vi "4155C Output-FPP.vi"(0 "VISA resource name in":refnum<visa-resource-name>="GPIB0::14::INSTR", 2 "Gate":T4={"Gate Start"=0.0, "Gate Stop"=2.0, "Gate Step"=1.0, "Gate Compliance"=0.0001, "Gate PComp"=0.0, "Range mode"=0, "Range"=6} {"Range" max=11 scale=0.0..11.0; "Range mode" items=["Auto", "Limited", "Fixed"]; "Gate PComp" format="%^.2e"; "Gate Compliance" format="%^.2e"; "Gate Step" format="%^.4e"; "Gate Stop" format="%^.4e"; "Gate Start" format="%^.4e"}, 3 "Drain":T5={"Drain Start"=0.0, "Drain Stop"=2.0, "Drain Compliance"=0.0001, "Drain Step (linear only)"=1.0, "Drain PComp"=0.0, "Range mode"=0, "Range"=6} {"Range" max=11 scale=0.0..11.0; "Range mode" items=["Auto", "Limited", "Fixed"]; "Drain PComp" format="%^.2e"; "Drain Step (linear only)" format="%^.4e"; "Drain Compliance" format="%^.2e"; "Drain Stop" format="%^.4e"; "Drain Start" format="%^.4e"}, 5 "Timings":T3={"integration time"=0, "Short/Long integration time"=0.00064, "hold time (sec)"=0.0, "delay time (sec)"=0.0, "Step Time (0 disables)"=0.0, "sweep method"=0, "Pulse period"=0.005, "Base voltage"=0.0, "Pulse width"=0.0005} {"Pulse width" min=0.0005 max=0.1 step=0.0001 format="%.4f"; "Base voltage" format="%^.4e"; "Pulse period" min=0.005 max=1.0 step=0.0001 format="%.4f"; "sweep method" items=["Continuous", "Pulsed"]; "Step Time (0 disables)" format="%.2f"; "delay time (sec)" format="%.4f"; "hold time (sec)" format="%.4f"; "Short/Long integration time" format="%^.0e"; "integration time" scale=0.0..2.0}, 6 "error in (no error)":errorcluster, 10 "sweep mode":u16(ring) items=["Single", "Double"], 12 "Panel controls":T2={"Emergency Stop"=refnum, "OutputGraph Max"=1e-05, "Text/Graph (text=false)"=FALSE} {"OutputGraph Max" format="%.2e"}) -> (16 "VD":dbl[](array[numeric]) format="%.2f", 17 "Outparams":T1={"V2 Start"=0.0, "V2 Step"=0.0, "Number of points"=1} {"V2 Step" format="%.2f"; "V2 Start" format="%^.4e"}, 20 "VISA Resource Name out":refnum<visa-resource-name>, 21 "Vprobe2":dbl[](array[numeric]) format="%.2f", 22 "ID":dbl[](array[numeric]) format="%.2f", 23 "IG":dbl[](array[numeric]) format="%.2f", 25 "Vprobe1":dbl[](array[numeric]) format="%.2f", 26 "error out":errorcluster)   [LabVIEW 2016]
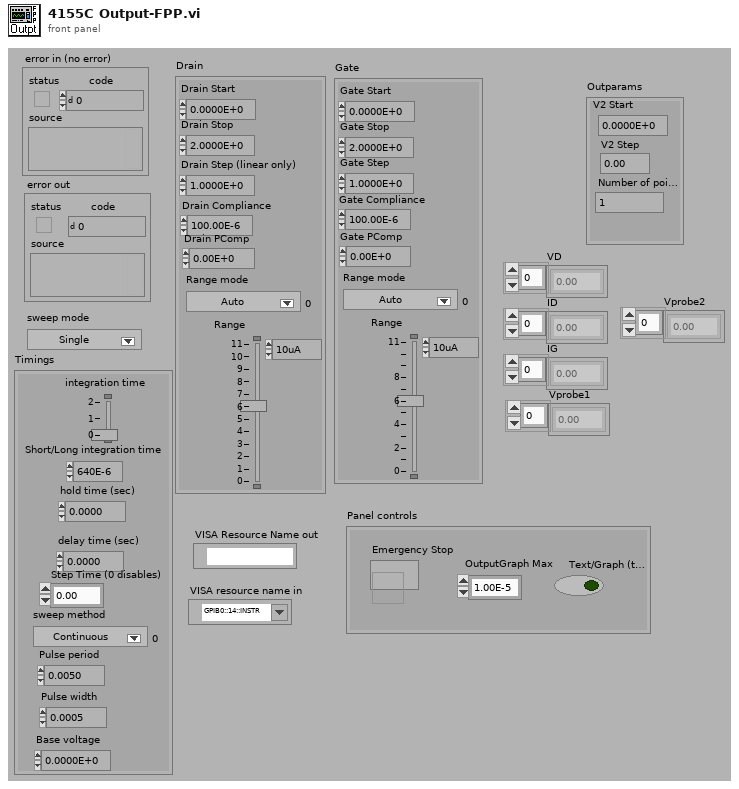
[diagram p1: front panel]
types:
  T1 = cluster{"V2 Start":dbl, "V2 Step":dbl, "Number of points":i32}
  T2 = cluster{"Emergency Stop":refnum<vi>, "OutputGraph Max":dbl, "Text/Graph (text=false)":bool}
  T3 = cluster{"integration time":u32, "Short/Long integration time":dbl, "hold time (sec)":dbl, "delay time (sec)":dbl, "Step Time (0 disables)":dbl, "sweep method":u16, "Pulse period":dbl, "Base voltage":dbl, "Pulse width":dbl}
  T4 = cluster{"Gate Start":dbl, "Gate Stop":dbl, "Gate Step":dbl, "Gate Compliance":dbl, "Gate PComp":dbl, "Range mode":u16, "Range":u8}
  T5 = cluster{"Drain Start":dbl, "Drain Stop":dbl, "Drain Compliance":dbl, "Drain Step (linear only)":dbl, "Drain PComp":dbl, "Range mode":u16, "Range":u8}
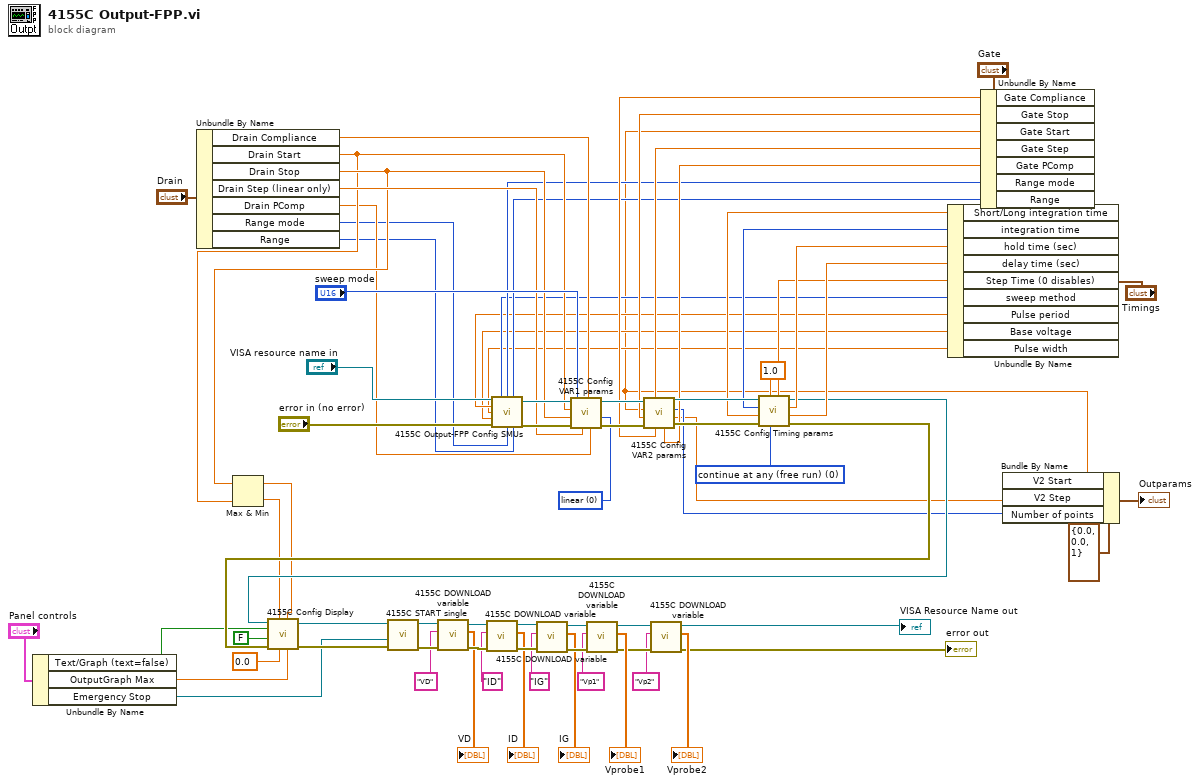
[diagram p0: block diagram]
diagram:
  w60 = u8 0 items=["continue at any (free run)", "stop at any abnorm", "stop at compliance"] ("stop condition (free run:0)")
  w57 = u16 0 items=["linear", "log 10", "log 25", "log 50"] ("sweep spacing (linear: 0)")
  n1 = Unbundle By Name("Panel controls") -> ("Text/Graph (text=false)"=w26:bool, "OutputGraph Max"=w25:dbl, "Emergency Stop"=w24:refnum<vi>)
  n2 = Unbundle By Name("Drain") -> ("Drain Compliance"=w44:dbl, "Drain Start"=w28:dbl, "Drain Stop"=w29:dbl, "Drain Step (linear only)"=w43:dbl, "Drain PComp"=w23:dbl, "Range mode"=w19:u16, "Range"=w18:u8)
  n3 = Max & Min(x=w29, y=w28) -> (max(x,y)=w1:dbl, min(x,y)=w2:dbl)
  n4 = Unbundle By Name("Timings") -> ("Short/Long integration time"=w62:dbl, "integration time"=w39:u32, "hold time (sec)"=w40:dbl, "delay time (sec)"=w41:dbl, "Step Time (0 disables)"=w36:dbl, "sweep method"=w17:u16, "Pulse period"=w16:dbl, "Base voltage"=w14:dbl, "Pulse width"=w15:dbl)
  n5 = Unbundle By Name("Gate") -> ("Gate Compliance"=w47:dbl, "Gate Stop"=w46:dbl, "Gate Start"=w9:dbl, "Gate Step"=w45:dbl, "Gate PComp"=w22:dbl, "Range mode"=w21:u16, "Range"=w20:u8)
  n6 = call "4155C Output-FPP Config SMUs.vi"("VISA resource name in"="VISA resource name in", "sweep method"=w17, "Gate mode"=w21, "Gate Range"=w20, "Pulse period"=w16, "Pulse width"=w15, "Base voltage"=w14, "error in (no error)"="error in (no error)", "Source/drain mode"=w19, "Source/drain Range"=w18) -> ("VISA Resource Name out"=w55:refnum<visa-resource-name>, "error out"=w54:errorcluster)  [unwired: 4 in]
  n7 = call "4155C Config VAR1 params.vi"("sweep spacing (linear: 0)"=w57, "power compliance (0 = OFF)"=w23, "compliance"=w44, "step (linear only)"=w43, "sweep mode"="sweep mode", "error in (no error)"=w54, "stop"=w29, "start"=w28, "VISA session"=w55) -> ("error out"=w58:errorcluster, "dup VISA resource name"=w59:refnum<visa-resource-name>)  [unwired: 1 out]
  n8 = call "4155C Config VAR2 params.vi"("power compliance (0 = OFF)"=w22, "compliance"=w47, "step"=w45, "error in (no error)"=w58, "stop"=w46, "start"=w9, "VISA session"=w59) -> ("error out"=w63:errorcluster, "Corrected Step"=w10:dbl, "Number of points"=w11:i32, "dup VISA resource name"=w64:refnum<visa-resource-name>)  [unwired: 1 in]
  n9 = call "4155C Config Timing params.vi"("delay time (sec)"=w41, "hold time (sec)"=w40, "Step Time (0 disables)"=w36, "stop condition (free run:0)"=w60, "wait time parameter"=1.0, "error in (no error)"=w63, "Short/Long integration time"=w62, "integration time"=w39, "VISA session"=w64) -> ("error out"=w33:errorcluster, "dup VISA resource name"=w32:refnum<visa-resource-name>)  [unwired: 1 in]
  n10 = call "4155C Config Display.vi"("Ymax"=w25, "Var1 Stop"=w1, "Ymin"=0.0, "Var1 Start"=w2, "error in (no error)"=w33, "Logarithmic"=FALSE, "SPA Display"=w26, "VISA session"=w32) -> ("error out"=w34:errorcluster, "dup VISA resource name"=w35:refnum<visa-resource-name>)  [unwired: 2 in]
  n11 = call "4155C START single.vi"("error in (no error)"=w34, "Emergency Stop"=w24, "VISA resource name in"=w35) -> ("error out"=w75:errorcluster, "VISA Resource Name out"=w76:refnum<visa-resource-name>)  [unwired: 3 in]
  n12 = call "4155C DOWNLOAD variable.vi"("error in (no error)"=w75, "Variable name"="VD", "VISA resource name in"=w76) -> ("error out"=w73:errorcluster, "Output data"=→"VD":dbl[], "VISA Resource Name out"=w72:refnum<visa-resource-name>)  [unwired: 2 in]
  n13 = call "4155C DOWNLOAD variable.vi"("error in (no error)"=w73, "Variable name"="ID", "VISA resource name in"=w72) -> ("error out"=w69:errorcluster, "Output data"=→"ID":dbl[], "VISA Resource Name out"=w70:refnum<visa-resource-name>)  [unwired: 2 in]
  n14 = call "4155C DOWNLOAD variable.vi"("error in (no error)"=w69, "Variable name"="IG", "VISA resource name in"=w70) -> ("error out"=w68:errorcluster, "Output data"=→"IG":dbl[], "VISA Resource Name out"=w67:refnum<visa-resource-name>)  [unwired: 2 in]
  n15 = call "4155C DOWNLOAD variable.vi"("error in (no error)"=w68, "Variable name"="Vp1", "VISA resource name in"=w67) -> ("error out"=w8:errorcluster, "Output data"=→"Vprobe1":dbl[], "VISA Resource Name out"=w7:refnum<visa-resource-name>)  [unwired: 2 in]
  n16 = call "4155C DOWNLOAD variable.vi"("error in (no error)"=w8, "Variable name"="Vp2", "VISA resource name in"=w7) -> ("error out"=→"error out":errorcluster, "Output data"=→"Vprobe2":dbl[], "VISA Resource Name out"=→"VISA Resource Name out":refnum<visa-resource-name>)  [unwired: 2 in]
  n17 = Bundle By Name(cluster=T1 {"V2 Start"=0.0, "V2 Step"=0.0, "Number of points"=1} ("Outparams"), "V2 Start"=w9, "V2 Step"=w10, "Number of points"=w11) -> (→"Outparams":T1)
